vi "Aula 1.vi"() -> ()   [LabVIEW 2024]
panel:
  out "I":i32
  out "Meter":dbl(knob) scale=0.0..10.0
  in  "N":i32
  out "element":dbl
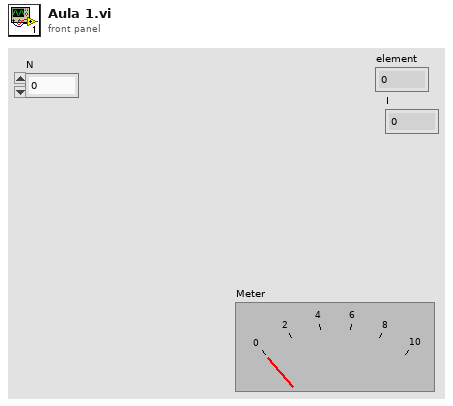
[diagram p1: front panel]
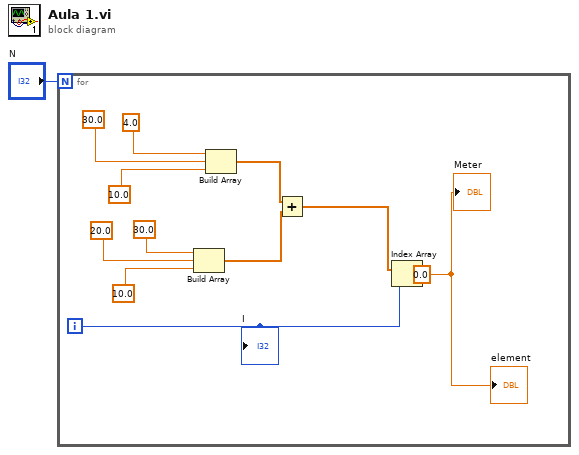
[diagram p0: block diagram]
diagram:
  n1 = for {
    N: "N" -> [_]
    i -> [w3]
    w2 = 0.0 ("element")
    n2 = Build Array(30.0 ("element"), 20.0 ("element"), 10.0 ("element")) -> (w5:dbl[])
    n3 = Build Array(4.0 ("element"), 30.0 ("element"), 10.0 ("element")) -> (w6:dbl[])
    n4 = Add(x=w6, y=w5) -> (x+y=w4:dbl[])
    n5 = Index Array(array=w4, index=w3) -> ()  [unwired: 1 out]
    "element" <- w2
    "Meter" <- w2
    "I" <- w3
  }
